vi "InitialConditions FGV.vi"(9 "Y0":dbl, 10 "X0":dbl, 11 "Enum":T1) -> (1 "Y0":dbl, 2 "X0":dbl)   [LabVIEW 2017, in "controllerLibrary.lvlib"]
uses:
  controllerLibrary.lvlib
  Controls/initial conditions control.ctl
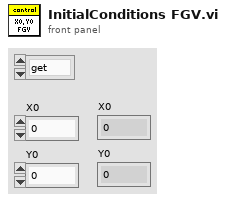
[diagram p1: front panel]
types:
  T1 = typedef "controllerLibrary.lvlib/initial conditions control.ctl" = enum16{"get", "set"}
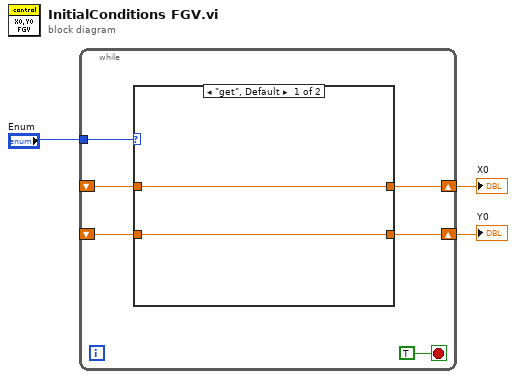
[diagram p0: block diagram]
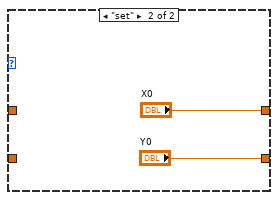
[diagram p2: hidden frame]
diagram:
  n1 = while {
    shift-right: [w7] -> w2
    shift-left: _ -> [w5]
    shift-right: [w6] -> w3
    shift-left: _ -> [w4]
    tunnel: "Enum" -> [w8]
    stop <- TRUE stop-if-true
    n2 = case shown="\"get\", Default" w8 {
      tunnel: [w11 "X0"] -> w7
      tunnel: [w10 "Y0"] -> w6
      tunnel: w5 -> [w11 _]
      tunnel: w4 -> [w10 _]
      frame "get", Default {
      }
      frame "set" {
      }
    }
  }
  "X0" <- w2
  "Y0" <- w3
